vi "Close.vi"(8 "error in (no error)":errorcluster, 11 "FW Arduino Control in":refnum<class "FW Arduino Control.lvclass">) -> (0 "error out":errorcluster, 3 "FW Arduino Control out":refnum<class "FW Arduino Control.lvclass">)   [LabVIEW 2021, in "FW Arduino Control.lvclass"]
uses:
  FW Arduino Control.lvclass
  FW Arduino Control.lvclass/FW Arduino Control.ctl
  Filter Wheel Object/Filter Wheel.lvclass
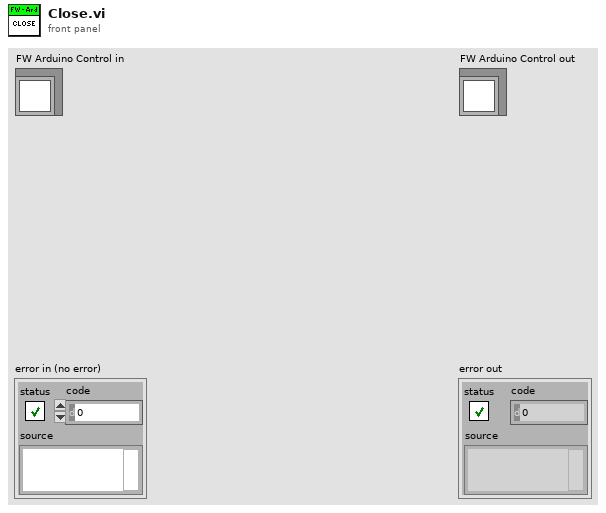
[diagram p1: front panel]
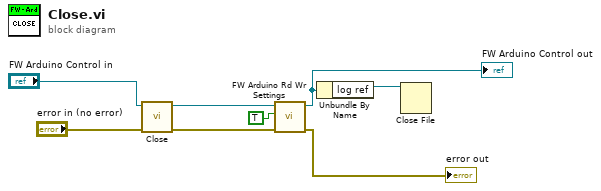
[diagram p0: block diagram]
diagram:
  n1 = call-parent "Close.vi"("error in (no error)"="error in (no error)", "Filter Wheel in"="FW Arduino Control in") -> ("error out"=w6:errorcluster, "Filter Wheel out"=w5:refnum<class "FW Arduino Control.lvclass">)  [unwired: 8 in]
  n2 = call "FW Arduino Rd Wr Settings.vi"("error in (no error)"=w6, "Write? (F:Read)"=TRUE, "Settings"=w5) -> ("error out"=→"error out":errorcluster, "Settings"=w2:refnum<class "FW Arduino Control.lvclass">)  [unwired: 7 in]
  "FW Arduino Control out" <- w2
  n3 = Unbundle By Name(w2) -> ("log ref"=w1:refnum<file>)
  n4 = Close File(refnum=w1) -> ()  [unwired: 1 in, 2 out]
